vi "Lab Panel V4.87.vi"() -> ()   [LabVIEW 2013] (continued)
              n211 = local read "LAB05 TEMP"() -> (w259:T12)
              n212 = Unbundle By Name(w259) -> ("T1 Live"=w258:dbl, "T1 Neut"=w257:dbl, "T2 Live"=w256:dbl, "T2 Neut"=w255:dbl)  [unwired: 2 out]
              n213 = local read "TEMP LA05"() -> (w260:T9)
              n214 = Bundle By Name(cluster=w260, "TL-1"=w258, "TN-1"=w257, "TL-2"=w256, "TN-2"=w255, "TL -1COUNT"=w253, "TN-1 COUNT"=w253, "TL-2 COUNT"=w253, "TN-2 COUNT"=w253) -> (w254:T9)
              n215 = local write "TEMP LA05"(w254) -> ()
            }
          }
        }
        frame #8 {
          # "enable front panel, all settings done"
          n216 = property on="Tab Control 2" class="TabCtl (strict)"("DisabledEnum"=T16."Enabled" ("Disabled")) -> ()  [unwired: 2 in, 2 out]
          n217 = property on="Tab Control 2" class="TabCtl (strict)"("Value"=0) -> ()  [unwired: 2 in, 2 out]
        }
        frame #9 {
          # "check network directory valid"
          n218 = while {
            stop <- w265 continue-if-true
            w263 = TRUE
            n219 = local read "Network Directory"() -> (w267:path)
            n220 = property on="Tab Control 2" class="TabCtl (strict)"("Value"=5) -> ()  [unwired: 2 in, 2 out]
            n221 = File/Directory Info(path=w267) -> (error out=w268:errorcluster)  [unwired: 1 in, 6 out]
            n222 = Unbundle(w268) -> ("status"=w265:bool)  [unwired: 2 out]
            n223 = case shown="True" w265 {
              frame False {
                n224 = local write "Message"("") -> ()
              }
              frame True {
                "Message" <- "NETWORK DIRECTORY NOT FOUND!!!!"
              }
            }
            n225 = property on="Message" class="Str"("Text.TextColor"=u32 16711680) -> ()  [unwired: 2 in, 2 out]
            n226 = property on="Network Directory" class="Path"("Blinking"=w263) -> ()  [unwired: 2 in, 2 out]
            n227 = property on="Message" class="Str"("Blinking"=w263) -> ()  [unwired: 2 in, 2 out]
          }
        }
        frame #10 {
          w271 = FALSE
          n228 = property on="Message" class="Str"("Blinking"=w271) -> ()  [unwired: 2 in, 2 out]
          n229 = property on="Network Directory" class="Path"("Blinking"=w271) -> ()  [unwired: 2 in, 2 out]
          n230 = property on="Tab Control 2" class="TabCtl (strict)"("Value"=0) -> ()  [unwired: 2 in, 2 out]
        }
      }
    }
    frame #2 {
      n231 = node-c288("loop  delay(mS)") -> (w275:T17)  [unwired: 3 in]
      n232 = timed-loop {
        timing: w275 -> [_]
        timing-out: [_] -> w274
        i -> [w297]
        stop <- "stop" stop-if-true
        n233 = node-c288() -> ()  [unwired: 1 in, 1 out]
        n234 = global write "Global display 1.vi" "stop disp"("stop") -> ()
        n235 = local read "SELECT LAB05-2"() -> (w277:T3)
        n236 = local read "SELECT LAB05-1"() -> (w278:T3)
        n237 = local read "SELECT LAB04-2"() -> (w279:T3)
        n238 = local read "SELECT LAB03-1"() -> (w282:T3)
        n239 = local read "SELECT LAB02-2"() -> (w283:T3)
        n240 = local read "SELECT LAB01-1"() -> (w286:T3)
        n241 = local read "SELECT LAB03-2"() -> (w281:T3)
        n242 = local read "SELECT LAB01-2"() -> (w285:T3)
        n243 = local read "SELECT LAB04-1"() -> (w280:T3)
        n244 = local read "SELECT LAB02-1"() -> (w284:T3)
        n245 = local read "run lab03-2"() -> (w291:bool)
        n246 = local read "run lab04-1"() -> (w290:bool)
        n247 = local read "run lab05-1"() -> (w288:bool)
        n248 = local read "run lab04-2"() -> (w289:bool)
        n249 = local read "run lab05-2"() -> (w287:bool)
        n250 = local read "run lab03-1"() -> (w292:bool)
        n251 = local read "run lab02-2"() -> (w293:bool)
        n252 = local read "run lab02-1"() -> (w294:bool)
        n253 = local read "run lab01-1"() -> (w296:bool)
        n254 = local read "run lab01-2"() -> (w295:bool)
        n255 = stacked-sequence {
          seq-local: [_ w359 _ _ _ _ _ _ _ _ _ _ _ _ _ _ _ _ _ _ _ _ _] -> [_ _ _ _ _ w2438 _ _ _ _ _ _ _ _ _ _ _ _ _ _ _ _ _]
          seq-local: [_ w358 _ _ _ _ _ _ _ _ _ _ _ _ _ _ _ _ _ _ _ _ _] -> [_ _ _ _ _ w2437 _ _ _ _ _ _ _ _ _ _ _ _ _ _ _ _ _]
          seq-local: [_ w345 _ _ _ _ _ _ _ _ _ _ _ _ _ _ _ _ _ _ _ _ _] -> [_ _ _ _ _ w2436 _ _ _ _ _ _ _ _ _ _ _ _ _ _ _ _ _]
          seq-local: [_ w344 _ _ _ _ _ _ _ _ _ _ _ _ _ _ _ _ _ _ _ _ _] -> [_ _ _ _ _ w2435 _ _ _ _ _ _ _ _ _ _ _ _ _ _ _ _ _]
          seq-local: [_ w343 _ _ _ _ _ _ _ _ _ _ _ _ _ _ _ _ _ _ _ _ _] -> [_ _ _ _ _ w2434 _ _ _ _ _ _ _ _ _ _ _ _ _ _ _ _ _]
          seq-local: [_ w342 _ _ _ _ _ _ _ _ _ _ _ _ _ _ _ _ _ _ _ _ _] -> [_ _ _ _ _ w2433 _ _ _ _ _ _ _ _ _ _ _ _ _ _ _ _ _]
          seq-local: [_ w341 _ _ _ _ _ _ _ _ _ _ _ _ _ _ _ _ _ _ _ _ _] -> [_ _ _ _ _ w2432 _ _ _ _ _ _ _ _ _ _ _ _ _ _ _ _ _]
          seq-local: [_ w340 _ _ _ _ _ _ _ _ _ _ _ _ _ _ _ _ _ _ _ _ _] -> [_ _ _ _ _ w2431 _ _ _ _ _ _ _ _ _ _ _ _ _ _ _ _ _]
          seq-local: [_ w339 _ _ _ _ _ _ _ _ _ _ _ _ _ _ _ _ _ _ _ _ _] -> [_ _ _ _ _ w2430 _ _ _ _ _ _ _ _ _ _ _ _ _ _ _ _ _]
          seq-local: [_ w338 _ _ _ _ _ _ _ _ _ _ _ _ _ _ _ _ _ _ _ _ _] -> [_ _ _ _ _ w2429 _ _ _ _ _ _ _ _ _ _ _ _ _ _ _ _ _]
          tunnel: w296 -> [_ _ w375 w621 w2028 w2458 w2773 w3260 _ _ _ _ w3671 _ w4628 _ _ w4913 w5216 w5398 _ _ _]
          tunnel: w295 -> [_ _ w374 w619 w2027 w2457 w2774 w3259 _ _ _ _ w3670 _ w4626 _ _ w4912 w5215 w5396 _ _ _]
          tunnel: w294 -> [_ _ w373 w617 w2026 w2456 w2772 w3258 _ _ _ _ w3669 _ w4624 _ _ w4911 w5214 w5395 _ _ _]
          tunnel: w293 -> [_ _ w372 w615 w2025 w2455 w2771 w3257 _ _ _ _ w3668 _ w4622 _ _ w4910 w5213 w5394 _ _ _]
          tunnel: w292 -> [_ _ w371 w613 w2024 w2454 w2770 w3256 _ _ _ _ w3667 _ w4620 _ _ w4909 w5212 w5393 _ _ _]
          tunnel: w291 -> [_ _ w370 w611 w2023 w2453 w2769 w3255 _ _ _ _ w3666 _ w4618 _ _ w4908 w5211 w5392 _ _ _]
          tunnel: w290 -> [_ _ w369 w609 w2022 w2452 w2768 w3254 _ _ _ _ w3665 _ w4616 _ _ w4907 w5210 w5391 _ _ _]
          tunnel: w289 -> [_ _ w368 w607 w2021 w2451 w2767 w3253 _ _ _ _ w3664 _ w4614 _ _ w4906 w5209 w5390 _ _ _]
          tunnel: w288 -> [_ _ w367 w605 w2020 w2450 w2766 w3252 _ _ _ _ w3663 _ w4612 _ _ w4905 w5208 w5389 _ _ _]
          tunnel: w287 -> [_ _ w366 w603 w2019 w2449 w2765 w3251 _ _ _ _ w3662 _ w4610 _ _ w4904 w5207 w5388 _ _ _]
          tunnel: w286 -> [_ _ _ w620 w2018 w2448 _ _ _ _ _ _ _ _ w4630 _ _ _ _ _ w5736 _ _]
          tunnel: w285 -> [_ _ _ w618 w2017 w2447 _ _ _ _ _ _ _ _ w4625 _ _ _ _ _ w5735 _ _]
          tunnel: w284 -> [_ _ _ w616 w2016 w2446 _ _ _ _ _ _ _ _ w4623 _ _ _ _ _ w5734 _ _]
          tunnel: w283 -> [_ _ _ w614 w2015 w2445 _ _ _ _ _ _ _ _ w4621 _ _ _ _ _ w5733 _ _]
          tunnel: w282 -> [_ _ _ w612 w2014 w2444 _ _ _ _ _ _ _ _ w4619 _ _ _ _ _ w5732 _ _]
          tunnel: w281 -> [_ _ _ w610 w2013 w2443 _ _ _ _ _ _ _ _ w4617 _ _ _ _ _ w5731 _ _]
          tunnel: w280 -> [_ _ _ w608 w2012 w2442 _ _ _ _ _ _ _ _ w4615 _ _ _ _ _ w5730 _ _]
          tunnel: w279 -> [_ _ _ w606 w2011 w2441 _ _ _ _ _ _ _ _ w4613 _ _ _ _ _ w5729 _ _]
          tunnel: w278 -> [_ _ _ w604 w2010 w2440 _ _ _ _ _ _ _ _ w4611 _ _ _ _ _ w5728 _ _]
          tunnel: w277 -> [_ _ _ w602 w2009 w2439 _ _ _ _ _ _ _ _ w4609 _ _ _ _ _ w5727 _ _]
          frame #0 {
            w301 = FALSE
            w306 = 0.5
            # "set up cycle control"
            n256 = local read "jig cycle"() -> (w305:dbl)
            n257 = Divide(x="JIG ON TIME (S)", y=w306) -> (x/y=→"on loops":dbl)
            n258 = Divide(x="JIG OFF TIME (S)", y=w306) -> (x/y=→"off loops":dbl)
            n259 = Increment(x=w305) -> (x+1=w304:dbl)
            n260 = local write "TEMP"(w301) -> ()
            n261 = local write "AI"(w301) -> ()
            n262 = local write "jig cycle"(w304) -> ()
            n263 = event shown="[1] \"ADMIN\": Value Change" {
              selector: _ -> [_ _]
              dyn-events: _ -> [_ _]
              timeout: 10 -> [_ _]
              event Timeout {
                n264 = event-data() -> ()  [unwired: 1 in, 3 out]
              }
              event "ADMIN": Value Change {
                n265 = event-data() -> ()  [unwired: 1 in, 6 out]
                n266 = stacked-sequence {
                  seq-local: [_ w310 _] -> [_ _ w311]
                  frame #0 {
                    n267 = global write "Global 1.vi" "password"("9999") -> ()
                  }
                  frame #1 {
                    n268 = call "sub vi - password 1.vi"() -> ("RESULT"=w310:bool)  [unwired: 11 in]
                  }
                  frame #2 {
                    w313 = FALSE
                    n269 = property on="Tab Control 2" class="TabCtl (strict)"() -> ("Pages"=w317:refnum<vi>[])  [unwired: 2 in, 2 out]
                    n270 = Select(t=TRUE, s=w311, f=w313) -> (s? t:f=w312:bool)
                    n271 = Index Array(array=w317, index=8) -> (element=w315:refnum<vi>)
                    n272 = property class="Page"(reference=w315, "PageVis"=w312) -> ()  [unwired: 1 in, 2 out]
                    n273 = local write "ADMIN"(w313) -> ()
                  }
                }
              }
            }
          }
          frame #1 {
            w355 = 60.0
            # "convert temperature rise minutes to cycles"
            n274 = local read "SET LAB05-2"() -> (w319:T5)
            n275 = local read "SET LAB05-1"() -> (w321:T5)
            n276 = local read "SET LAB04-2"() -> (w323:T5)
            n277 = local read "SET LAB01-1"() -> (w337:T5)
            n278 = local read "SET LAB01-2"() -> (w335:T5)
            n279 = local read "SET LAB02-2"() -> (w331:T5)
            n280 = local read "SET LAB04-1"() -> (w325:T5)
            n281 = local read "SET LAB03-1"() -> (w329:T5)
            n282 = local read "SET LAB03-2"() -> (w327:T5)
            n283 = local read "SET LAB02-1"() -> (w333:T5)
            n284 = local read "JIG OFF TIME (S)"() -> (w360:dbl)
            n285 = local read "JIG ON TIME (S)"() -> (w361:dbl)
            n286 = Unbundle(w319) -> ("T-RISE mins"=w318:dbl)  [unwired: 4 out]
            n287 = Unbundle(w321) -> ("T-RISE mins"=w320:dbl)  [unwired: 4 out]
            n288 = Unbundle(w337) -> ("T-RISE mins"=w336:dbl)  [unwired: 4 out]
            n289 = Unbundle(w323) -> ("T-RISE mins"=w322:dbl)  [unwired: 4 out]
            n290 = Unbundle(w335) -> ("T-RISE mins"=w334:dbl)  [unwired: 4 out]
            n291 = Unbundle(w333) -> ("T-RISE mins"=w332:dbl)  [unwired: 4 out]
            n292 = Unbundle(w325) -> ("T-RISE mins"=w324:dbl)  [unwired: 4 out]
            n293 = Unbundle(w331) -> ("T-RISE mins"=w330:dbl)  [unwired: 4 out]
            n294 = Unbundle(w327) -> ("T-RISE mins"=w326:dbl)  [unwired: 4 out]
            n295 = Unbundle(w329) -> ("T-RISE mins"=w328:dbl)  [unwired: 4 out]
            n296 = Add(x=w361, y=w360) -> (x+y=w354:dbl)
            n297 = Multiply(x=w355, y=w326) -> (x*y=w350:dbl)
            n298 = Multiply(x=w355, y=w324) -> (x*y=w349:dbl)
            n299 = Multiply(x=w355, y=w322) -> (x*y=w348:dbl)
            n300 = Multiply(x=w355, y=w320) -> (x*y=w347:dbl)
            n301 = Multiply(x=w355, y=w318) -> (x*y=w346:dbl)
            n302 = Multiply(x=w355, y=w334) -> (x*y=w356:dbl)
            n303 = Multiply(x=w355, y=w328) -> (x*y=w351:dbl)
            n304 = Multiply(x=w355, y=w336) -> (x*y=w357:dbl)
            n305 = Multiply(x=w355, y=w332) -> (x*y=w353:dbl)
            n306 = Multiply(x=w355, y=w330) -> (x*y=w352:dbl)
            n307 = Divide(x=w347, y=w354) -> (x/y=w339:dbl)
            n308 = Divide(x=w348, y=w354) -> (x/y=w340:dbl)
            n309 = Divide(x=w349, y=w354) -> (x/y=w341:dbl)
            n310 = Divide(x=w346, y=w354) -> (x/y=w338:dbl)
            n311 = Divide(x=w351, y=w354) -> (x/y=w343:dbl)
            n312 = Divide(x=w357, y=w354) -> (x/y=w359:dbl)
            n313 = Divide(x=w356, y=w354) -> (x/y=w358:dbl)
            n314 = Divide(x=w353, y=w354) -> (x/y=w345:dbl)
            n315 = Divide(x=w352, y=w354) -> (x/y=w344:dbl)
            n316 = Divide(x=w350, y=w354) -> (x/y=w342:dbl)
          }
          frame #2 {
            # "control cycle loops"
            n317 = local read "JIG OFF TIME (S)"() -> (w364:dbl)
            n318 = local read "JIG ON TIME (S)"() -> (w363:dbl)
            n319 = local read "jig cycle"() -> (w377:dbl)
            n320 = local read "on loops"() -> (w379:dbl)
            n321 = local read "off loops"() -> (w378:dbl)
            n322 = Add(x=w364, y=w363) -> (x+y=w362:dbl)
            n323 = Add(x=w379, y=w378) -> (x+y=w365:dbl)
            n324 = Greater Or Equal?(x=w377, y=w365) -> (x >= y?=w376:bool)
            n325 = case shown="True" w376 {
              tunnel: w375 -> [_ w412]
              tunnel: w374 -> [_ w411]
              tunnel: w373 -> [_ w410]
              tunnel: w372 -> [_ w409]
              tunnel: w371 -> [_ w408]
              tunnel: w370 -> [_ w407]
              tunnel: w369 -> [_ w406]
              tunnel: w368 -> [_ w405]
              tunnel: w367 -> [_ w404]
              tunnel: w366 -> [_ w403]
              tunnel: w362 -> [_ w402]
              frame False {
              }
              frame True {
                # "increment cycle value and convert cycles to minutes for temp rise"
                n326 = stacked-sequence {
                  frame #0 {
                    n327 = local read "PANEL #"() -> (w415:dbl)
                    n328 = Increment(x=w415) -> (x+1=w414:dbl)
                    n329 = local write "PANEL #"(w414) -> ()
                  }
                  frame #1 {
                    n330 = local read "PANEL #"() -> (w416:dbl)
                    n331 = Greater?(x=w416, y=5) -> (0:w418:bool)
                    n332 = case shown="True" w418 {
                      frame False {
                      }
                      frame True {
                        n333 = local write "PANEL #"(1) -> ()
                      }
                    }
                  }
                }
                n334 = local read "JIG RELAY CYCLES"() -> (w401:T8)
                n335 = Unbundle By Name(w401) -> ("LAB01-1"=w399:dbl, "LAB01-2"=w397:dbl, "LAB02-1"=w395:dbl, "LAB02-2"=w393:dbl, "LAB03-1"=w391:dbl, "LAB03-2"=w389:dbl, "LAB04-1"=w387:dbl, "LAB04-2"=w385:dbl, "LAB05-1"=w383:dbl, "LAB05-2"=w381:dbl)
                n336 = stacked-sequence {
                  tunnel: w412 -> [w430 _ _ _ _ _ _ _ _ _]
                  tunnel: w411 -> [_ w447 _ _ _ _ _ _ _ _]
                  tunnel: w410 -> [_ _ w464 _ _ _ _ _ _ _]
                  tunnel: w409 -> [_ _ _ w481 _ _ _ _ _ _]
                  tunnel: w408 -> [_ _ _ _ w498 _ _ _ _ _]
                  tunnel: w407 -> [_ _ _ _ _ w515 _ _ _ _]
                  tunnel: w406 -> [_ _ _ _ _ _ w532 _ _ _]
                  tunnel: w405 -> [_ _ _ _ _ _ _ w549 _ _]
                  tunnel: w404 -> [_ _ _ _ _ _ _ _ w566 _]
                  tunnel: w403 -> [_ _ _ _ _ _ _ _ _ w583]
                  tunnel: w402 -> [w427 w444 w461 w478 w495 w512 w529 w546 w563 w580]
                  tunnel: w399 -> [w421 _ _ _ _ _ _ _ _ _]
                  tunnel: [w420 _ _ _ _ _ _ _ _ _] -> w398
                  tunnel: w397 -> [_ w438 _ _ _ _ _ _ _ _]
                  tunnel: [_ w437 _ _ _ _ _ _ _ _] -> w396
                  tunnel: w395 -> [_ _ w455 _ _ _ _ _ _ _]
                  tunnel: [_ _ w454 _ _ _ _ _ _ _] -> w394
                  tunnel: w393 -> [_ _ _ w472 _ _ _ _ _ _]
                  tunnel: [_ _ _ w471 _ _ _ _ _ _] -> w392
                  tunnel: w391 -> [_ _ _ _ w489 _ _ _ _ _]
                  tunnel: [_ _ _ _ w488 _ _ _ _ _] -> w390
                  tunnel: w389 -> [_ _ _ _ _ w506 _ _ _ _]
                  tunnel: [_ _ _ _ _ w505 _ _ _ _] -> w388
                  tunnel: w387 -> [_ _ _ _ _ _ w523 _ _ _]
                  tunnel: [_ _ _ _ _ _ w522 _ _ _] -> w386
                  tunnel: w385 -> [_ _ _ _ _ _ _ w540 _ _]
                  tunnel: [_ _ _ _ _ _ _ w539 _ _] -> w384
                  tunnel: w383 -> [_ _ _ _ _ _ _ _ w557 _]
                  tunnel: [_ _ _ _ _ _ _ _ w556 _] -> w382
                  tunnel: w381 -> [_ _ _ _ _ _ _ _ _ w574]
                  tunnel: [_ _ _ _ _ _ _ _ _ w573] -> w380
                  frame #0 {
                    n337 = local read "DISP LAB01-1"() -> (w425:T4)
                    n338 = Unbundle(w425) -> ("CYCLE"=w426:dbl)  [unwired: 2 out]
                    n339 = case shown="True" w430 {
                      tunnel: w426 -> [w432 w436]
                      tunnel: [w432 w435] -> w424
                      tunnel: w421 -> [w431 w434]
                      tunnel: [w431 w433] -> w420
                      frame False {
                      }
                      frame True {
                        n340 = Increment(x=w434) -> (x+1=w433:dbl)
                        n341 = Increment(x=w436) -> (x+1=w435:dbl)
                      }
                    }
                    n342 = Multiply(x=w424, y=w427) -> (x*y=w428:dbl)
                    n343 = Divide(x=w428, y=60.0) -> (x/y=w423:dbl)
                    n344 = Bundle(cluster=w425, "CYCLE"=w424, "MINS"=w423) -> (w422:T4)  [unwired: 1 in]
                    n345 = local write "DISP LAB01-1"(w422) -> ()
                  }
                  frame #1 {
                    n346 = local read "DISP LAB01-2"() -> (w442:T4)
                    n347 = Unbundle(w442) -> ("CYCLE"=w443:dbl)  [unwired: 2 out]
                    n348 = case shown="True" w447 {
                      tunnel: w443 -> [w449 w453]
                      tunnel: [w449 w452] -> w440
                      tunnel: w438 -> [w448 w451]
                      tunnel: [w448 w450] -> w437
                      frame False {
                      }
                      frame True {
                        n349 = Increment(x=w451) -> (x+1=w450:dbl)
                        n350 = Increment(x=w453) -> (x+1=w452:dbl)
                      }
                    }
                    n351 = Multiply(x=w440, y=w444) -> (x*y=w445:dbl)
                    n352 = Divide(x=w445, y=60.0) -> (x/y=w439:dbl)
                    n353 = Bundle(cluster=w442, "CYCLE"=w440, "MINS"=w439) -> (w441:T4)  [unwired: 1 in]
                    n354 = local write "DISP LAB01-2"(w441) -> ()
                  }
                  frame #2 {
                    n355 = local read "DISP LAB02-1"() -> (w459:T4)
                    n356 = Unbundle(w459) -> ("CYCLE"=w460:dbl)  [unwired: 2 out]
                    n357 = case shown="True" w464 {
                      tunnel: [w466 w470] -> w457
                      tunnel: w460 -> [w466 w469]
                      tunnel: w455 -> [w465 w468]
                      tunnel: [w465 w467] -> w454
                      frame False {
                      }
                      frame True {
                        n358 = Increment(x=w468) -> (x+1=w467:dbl)
                        n359 = Increment(x=w469) -> (x+1=w470:dbl)
                      }
                    }
                    n360 = Multiply(x=w457, y=w461) -> (x*y=w462:dbl)
                    n361 = Divide(x=w462, y=60.0) -> (x/y=w456:dbl)
                    n362 = Bundle(cluster=w459, "CYCLE"=w457, "MINS"=w456) -> (w458:T4)  [unwired: 1 in]
                    n363 = local write "DISP LAB02-1"(w458) -> ()
                  }
                  frame #3 {
                    n364 = local read "DISP LAB02-2"() -> (w476:T4)
                    n365 = Unbundle(w476) -> ("CYCLE"=w477:dbl)  [unwired: 2 out]
                    n366 = case shown="True" w481 {
                      tunnel: [w483 w487] -> w475
                      tunnel: w477 -> [w483 w486]
                      tunnel: w472 -> [w482 w485]
                      tunnel: [w482 w484] -> w471
                      frame False {
                      }
                      frame True {
                        n367 = Increment(x=w485) -> (x+1=w484:dbl)
                        n368 = Increment(x=w486) -> (x+1=w487:dbl)
                      }
                    }
                    n369 = Multiply(x=w475, y=w478) -> (x*y=w479:dbl)
                    n370 = Divide(x=w479, y=60.0) -> (x/y=w474:dbl)
                    n371 = Bundle(cluster=w476, "CYCLE"=w475, "MINS"=w474) -> (w473:T4)  [unwired: 1 in]
                    n372 = local write "DISP LAB02-2"(w473) -> ()
                  }
                  frame #4 {
                    n373 = local read "DISP LAB03-1"() -> (w493:T4)
                    n374 = Unbundle(w493) -> ("CYCLE"=w494:dbl)  [unwired: 2 out]
                    n375 = case shown="True" w498 {
                      tunnel: [w500 w504] -> w490
                      tunnel: w494 -> [w500 w503]
                      tunnel: w489 -> [w499 w502]
                      tunnel: [w499 w501] -> w488
                      frame False {
                      }
                      frame True {
                        n376 = Increment(x=w502) -> (x+1=w501:dbl)
                        n377 = Increment(x=w503) -> (x+1=w504:dbl)
                      }
                    }
                    n378 = Multiply(x=w490, y=w495) -> (x*y=w496:dbl)
                    n379 = Divide(x=w496, y=60.0) -> (x/y=w491:dbl)
                    n380 = Bundle(cluster=w493, "CYCLE"=w490, "MINS"=w491) -> (w492:T4)  [unwired: 1 in]
                    n381 = local write "DISP LAB03-1"(w492) -> ()
                  }
                  frame #5 {
                    n382 = local read "DISP LAB03-2"() -> (w510:T4)
                    n383 = Unbundle(w510) -> ("CYCLE"=w511:dbl)  [unwired: 2 out]
                    n384 = case shown="True" w515 {
                      tunnel: [w517 w521] -> w509
                      tunnel: w511 -> [w517 w520]
                      tunnel: w506 -> [w516 w519]
                      tunnel: [w516 w518] -> w505
                      frame False {
                      }
                      frame True {
                        n385 = Increment(x=w519) -> (x+1=w518:dbl)
                        n386 = Increment(x=w520) -> (x+1=w521:dbl)
                      }
                    }
                    n387 = Multiply(x=w509, y=w512) -> (x*y=w513:dbl)
                    n388 = Divide(x=w513, y=60.0) -> (x/y=w508:dbl)
                    n389 = Bundle(cluster=w510, "CYCLE"=w509, "MINS"=w508) -> (w507:T4)  [unwired: 1 in]
                    n390 = local write "DISP LAB03-2"(w507) -> ()
                  }
                  frame #6 {
                    n391 = local read "DISP LAB04-1"() -> (w527:T4)
                    n392 = Unbundle(w527) -> ("CYCLE"=w528:dbl)  [unwired: 2 out]
                    n393 = case shown="True" w532 {
                      tunnel: [w534 w538] -> w525
                      tunnel: w528 -> [w534 w537]
                      tunnel: w523 -> [w533 w536]
                      tunnel: [w533 w535] -> w522
                      frame False {
                      }
                      frame True {
                        n394 = Increment(x=w536) -> (x+1=w535:dbl)
                        n395 = Increment(x=w537) -> (x+1=w538:dbl)
                      }
                    }
                    n396 = Multiply(x=w525, y=w529) -> (x*y=w530:dbl)
                    n397 = Divide(x=w530, y=60.0) -> (x/y=w524:dbl)
                    n398 = Bundle(cluster=w527, "CYCLE"=w525, "MINS"=w524) -> (w526:T4)  [unwired: 1 in]
                    n399 = local write "DISP LAB04-1"(w526) -> ()
                  }
                  frame #7 {
                    n400 = local read "DISP LAB04-2"() -> (w544:T4)
                    n401 = Unbundle(w544) -> ("CYCLE"=w545:dbl)  [unwired: 2 out]
                    n402 = case shown="True" w549 {
                      tunnel: [w551 w555] -> w542
                      tunnel: w545 -> [w551 w554]
                      tunnel: w540 -> [w550 w553]
                      tunnel: [w550 w552] -> w539
                      frame False {
                      }
                      frame True {
                        n403 = Increment(x=w553) -> (x+1=w552:dbl)
                        n404 = Increment(x=w554) -> (x+1=w555:dbl)
                      }
                    }
                    n405 = Multiply(x=w542, y=w546) -> (x*y=w548:dbl)
                    n406 = Divide(x=w548, y=60.0) -> (x/y=w541:dbl)
                    n407 = Bundle(cluster=w544, "CYCLE"=w542, "MINS"=w541) -> (w543:T4)  [unwired: 1 in]
                    n408 = local write "DISP LAB04-2"(w543) -> ()
                  }
                  frame #8 {
                    n409 = local read "DISP LAB05-1"() -> (w561:T4)
                    n410 = Unbundle(w561) -> ("CYCLE"=w562:dbl)  [unwired: 2 out]
                    n411 = case shown="True" w566 {
                      tunnel: [w568 w572] -> w559
                      tunnel: w562 -> [w568 w571]
                      tunnel: w557 -> [w567 w570]
                      tunnel: [w567 w569] -> w556
                      frame False {
                      }
                      frame True {
                        n412 = Increment(x=w570) -> (x+1=w569:dbl)
                        n413 = Increment(x=w571) -> (x+1=w572:dbl)
                      }
                    }
                    n414 = Multiply(x=w559, y=w563) -> (x*y=w564:dbl)
                    n415 = Divide(x=w564, y=60.0) -> (x/y=w558:dbl)
                    n416 = Bundle(cluster=w561, "CYCLE"=w559, "MINS"=w558) -> (w560:T4)  [unwired: 1 in]
                    n417 = local write "DISP LAB05-1"(w560) -> ()
                  }
                  frame #9 {
                    n418 = local read "DISP LAB05-2"() -> (w579:T4)
                    n419 = Unbundle(w579) -> ("CYCLE"=w578:dbl)  [unwired: 2 out]
                    n420 = case shown="True" w583 {
                      tunnel: [w585 w589] -> w577
                      tunnel: w578 -> [w585 w588]
                      tunnel: w574 -> [w584 w587]
                      tunnel: [w584 w586] -> w573
                      frame False {
                      }
                      frame True {
                        n421 = Increment(x=w587) -> (x+1=w586:dbl)
                        n422 = Increment(x=w588) -> (x+1=w589:dbl)
                      }
                    }
                    n423 = Multiply(x=w577, y=w580) -> (x*y=w581:dbl)
                    n424 = Divide(x=w581, y=60.0) -> (x/y=w576:dbl)
                    n425 = Bundle(cluster=w579, "CYCLE"=w577, "MINS"=w576) -> (w575:T4)  [unwired: 1 in]
                    n426 = local write "DISP LAB05-2"(w575) -> ()
                  }
                }
                n427 = local write "jig cycle"(0) -> ()
                n428 = Bundle By Name(cluster=w401, "LAB01-1"=w398, "LAB01-2"=w396, "LAB02-1"=w394, "LAB02-2"=w392, "LAB03-1"=w390, "LAB03-2"=w388, "LAB04-1"=w386, "LAB04-2"=w384, "LAB05-1"=w382, "LAB05-2"=w380) -> (w400:T8)
                n429 = local write "JIG RELAY CYCLES"(w400) -> ()
              }
            }
          }
          frame #3 {
            # "START & STOP test RUN switch change, start test if true and stop test if false"
            n430 = Get Date/Time In Seconds() -> (seconds since 1Jan1904=w600:timestamp)
            n431 = local read "C drive data root dir"() -> (w593:path)
            n432 = Format Date/Time String(time format string (%c)="%b\\%a%d", seconds (now)=w600) -> (date/time string=w624:string)  [unwired: 1 in]
            n433 = Format Date/Time String(time format string (%c)="%H%M", seconds (now)=w600) -> (date/time string=w622:string)  [unwired: 1 in]
            n434 = Format Date/Time String(time format string (%c)="LabPanel%Y", seconds (now)=w600) -> (date/time string=w599:string)  [unwired: 1 in]
            n435 = Path To String(path=w593) -> (string=w596:string)
            n436 = global write "Global 1.vi" "C drive root path"(w593) -> ()
            n437 = Concatenate Strings(w596, "\\") -> (w594:string)
            n438 = event shown="[10] \"RUN LAB05-2\": Value Change" {
              selector: _ -> [_ _ _ _ _ _ _ _ _ _ _]
              dyn-events: _ -> [_ _ _ _ _ _ _ _ _ _ _]
              timeout: 10 -> [_ _ _ _ _ _ _ _ _ _ _]
              tunnel: w594 -> [_ w636 w774 w913 w1051 w1189 w1327 w1465 w1603 w1741 w1880]
              tunnel: w624 -> [_ w635 w773 w912 w1050 w1188 w1326 w1464 w1602 w1740 w1879]
              tunnel: w622 -> [_ w633 w772 w911 w1049 w1187 w1325 w1463 w1601 w1739 w1878]
              tunnel: w620 -> [_ w634 _ _ _ _ _ _ _ _ _]
              tunnel: w621 -> [_ _ _ _ _ _ _ _ _ _ _]
              tunnel: w619 -> [_ _ _ _ _ _ _ _ _ _ _]
              tunnel: w618 -> [_ _ w771 _ _ _ _ _ _ _ _]
              tunnel: w617 -> [_ _ _ _ _ _ _ _ _ _ _]
              tunnel: w616 -> [_ _ _ w910 _ _ _ _ _ _ _]
              tunnel: w615 -> [_ _ _ _ _ _ _ _ _ _ _]
              tunnel: w614 -> [_ _ _ _ w1048 _ _ _ _ _ _]
              tunnel: w613 -> [_ _ _ _ _ _ _ _ _ _ _]
              tunnel: w612 -> [_ _ _ _ _ w1186 _ _ _ _ _]
              tunnel: w611 -> [_ _ _ _ _ _ _ _ _ _ _]
              tunnel: w610 -> [_ _ _ _ _ _ w1324 _ _ _ _]
              tunnel: w609 -> [_ _ _ _ _ _ _ _ _ _ _]
              tunnel: w608 -> [_ _ _ _ _ _ _ w1462 _ _ _]
              tunnel: w607 -> [_ _ _ _ _ _ _ _ _ _ _]
              tunnel: w606 -> [_ _ _ _ _ _ _ _ w1600 _ _]
              tunnel: w605 -> [_ _ _ _ _ _ _ _ _ _ _]
              tunnel: w604 -> [_ _ _ _ _ _ _ _ _ w1738 _]
              tunnel: w603 -> [_ _ _ _ _ _ _ _ _ _ _]
              tunnel: w602 -> [_ _ _ _ _ _ _ _ _ _ w1877]
              tunnel: w599 -> [_ w632 w770 w909 w1047 w1185 w1323 w1461 w1599 w1737 w1876]
              tunnel: [_ w631 w769 w908 w1046 w1184 w1322 w1460 w1598 w1736 w1875] -> w597
              tunnel: "RESET CYCLES TO ZERO?" -> [_ w630 w767 w906 w1044 w1182 w1320 w1458 w1596 w1734 w1873]
              tunnel: "YES" -> [_ w629 w766 w905 w1043 w1181 w1319 w1457 w1595 w1733 w1872]
              tunnel: "NO" -> [_ w628 w765 w904 w1042 w1180 w1318 w1456 w1594 w1732 w1871]
              event Timeout {
                n439 = event-data() -> ()  [unwired: 1 in, 3 out]
              }
              event "RUN LAB01-1": Value Change {
                n440 = event-data() -> ("NewVal"=w626:bool)  [unwired: 1 in, 5 out]
                n441 = local read "SIG LAB01-1"() -> (w627:T2)
                n442 = local write "run lab01-1"(w626) -> ()
                n443 = case shown="True" w626 {
                  tunnel: w636 -> [_ w673]
                  tunnel: w635 -> [_ w672]
                  tunnel: w634 -> [w638 w671]
                  tunnel: w633 -> [_ w670]
                  tunnel: w632 -> [_ w669]
                  tunnel: [w637 w668] -> w631
                  tunnel: w630 -> [_ w667]
                  tunnel: w629 -> [_ w666]
                  tunnel: w628 -> [_ w665]
                  tunnel: w627 -> [_ w664]
                  frame False {
                    # "stop test"
                    n444 = stacked-sequence {
                      tunnel: w638 -> [_ w650 _]
                      tunnel: [_ w642 _] -> w637
                      frame #0 {
                        n445 = local read "DISP LAB01-1"() -> (w641:T4)
                        n446 = Bundle(cluster=w641, "STATUS"="STOP") -> (w639:T4)  [unwired: 2 in]
                        n447 = local write "DISP LAB01-1"(w639) -> ()
                      }
                      frame #1 {
                        n448 = local read "DISP LAB01-1"() -> (w649:T4)
                        n449 = Unbundle(w649) -> ("CYCLE"=w647:dbl, "MINS"=w648:dbl)  [unwired: 1 out]
                        n450 = case shown="\"CYCLE TEST\"" w650 {
                          tunnel: w648 -> [_ _ w657]
                          tunnel: w647 -> [w655 w656 _]
                          tunnel: [w655 w656 w657] -> w646
                          frame "CHART TEST", Default {
                          }
                          frame "CYCLE TEST" {
                          }
                          frame "T-RISE TEST" {
                          }
                        }
                        n451 = local read "TDMS LAB01-1"() -> (w654:refnum<k34>)
                        n452 = Build Array("STOPPED") -> (w651:string[])
                        n453 = Build Array(w646) -> (w645:dbl[])
                        n454 = TDMS Write(0:w654, 5:"TEST RESULT", 7:w651, 9:w645) -> (4:w643:refnum<k34>, 15:w644:errorcluster)  [unwired: 2 in, 2 out]
                        n455 = TDMS Close(8:w644, 11:w643) -> (0:w642:errorcluster)  [unwired: 1 out]
                      }
                      frame #2 {
                        n456 = stacked-sequence {
                          tunnel: "LAB01-1" -> [w660 w662]
                          frame #0 {
                            n457 = call "sub vi - defrag tdms v1.vi"("panel id"=w660) -> ("error out"=w659:errorcluster)  [unwired: 10 in]
                            n458 = local write "data file error"(w659) -> ()
                          }
                          frame #1 {
                            n459 = call "Save data file to network drive v2.vi"("panel id"=w662) -> ("network file save error"=w661:errorcluster)  [unwired: 9 in, 1 out]
                            n460 = local write "RESULT LAB01-1"(FALSE) -> ()
                            n461 = local write "data file error"(w661) -> ()
                          }
                        }
                      }
                    }
                  }
                  frame True {
                    n462 = stacked-sequence {
                      seq-local: [w675 _] -> [_ w678]
                      tunnel: w673 -> [_ w688]
                      tunnel: w672 -> [_ w687]
                      tunnel: w671 -> [_ w686]
                      tunnel: w670 -> [_ w685]
                      tunnel: w669 -> [_ w684]
                      tunnel: [_ w683] -> w668
                      tunnel: w667 -> [_ w682]
                      tunnel: w666 -> [_ w681]
                      tunnel: w665 -> [_ w680]
                      tunnel: w664 -> [w677 w679]
                      frame #0 {
                        n463 = Unbundle(w677) -> ("AMPS"=w676:dbl)  [unwired: 4 out]
                        n464 = call "Check For Amps on v1.vi"("ID"="LAB01-1", "amps"=w676) -> ("amps"=w675:bool)  [unwired: 9 in]
                      }
                      frame #1 {
                        n465 = case shown="True" w678 {
                          tunnel: w688 -> [_ w700]
                          tunnel: w687 -> [_ w699]
                          tunnel: w686 -> [_ w698]
                          tunnel: w685 -> [_ w697]
                          tunnel: w684 -> [_ w696]
                          tunnel: [errorcluster {"status"=FALSE, "code"=0, "source"=""} ("error out") w695] -> w683
                          tunnel: w682 -> [_ w694]
                          tunnel: w681 -> [_ w693]
                          tunnel: w680 -> [_ w692]
                          tunnel: w679 -> [_ w691]
                          frame False {
                            w689 = FALSE
                            n466 = local write "RUN LAB01-1"(w689) -> ()
                            n467 = local write "run lab01-1"(w689) -> ()
                          }
                          frame True {
                            n468 = stacked-sequence {
                              seq-local: [w701 _ _ _ _] -> [_ w722 _ _ _]
                              tunnel: w700 -> [w706 _ _ _ _]
                              tunnel: w699 -> [w702 _ _ _ _]
                              tunnel: w698 -> [w716 _ _ _ _]
                              tunnel: w697 -> [w709 _ _ _ _]
                              tunnel: w696 -> [w704 _ _ _ _]
                              tunnel: [_ w723 _ _ _] -> w695
                              tunnel: w694 -> [_ _ _ w744 _]
                              tunnel: w693 -> [_ _ _ w754 _]
                              tunnel: w692 -> [_ _ _ w753 _]
                              tunnel: w691 -> [_ _ _ _ w760]
                              frame #0 {
                                w703 = "\\"
                                n469 = case shown="\"CHART TEST\", Default" w716 {
                                tunnel: ["L01-1-CHART TEST-" "L01-1-CYCLE TEST-" "L01-1-T-RISE TEST-"] -> w712
                                frame "CHART TEST", Default {
                                }
                                frame "CYCLE TEST" {
                                }
                                frame "T-RISE TEST" {
                                }
                                }
                                n470 = local read "SET LAB01-1"() -> (w711:T5)
                                n471 = Unbundle(w711) -> ("DESCRIPTION"=w710:string)  [unwired: 4 out]
                                n472 = Concatenate Strings(w706, "\\", w704, w703, w702, w703) -> (w713:string)
                                n473 = String To Path(string=w713) -> (path=w715:path)
                                n474 = Concatenate Strings(w713, w712, w710, "-", w709, ".tdms") -> (w701:string)
                                n475 = Create Folder(path (use dialog)=w715) -> (error out=w714:errorcluster)  [unwired: 2 in, 2 out]
                                n476 = call <vilib>:"Clear Errors.vi"("error in (no error)"=w714) -> ()  [unwired: 6 in, 1 out]
                                n477 = global write "Global 1.vi" "LAB01-1 FILE"(w701) -> ()
                              }
                              frame #1 {
                                (unwired) FALSE
                                n478 = String To Path(string=w722) -> (path=w720:path)
                                n479 = TDMS Open(6:FALSE, 10:T20."create or replace" ("operation (0:open)"), 11:w720) -> (0:w723:errorcluster, 3:→"TDMS LAB01-1":refnum<k34>)  [unwired: 4 in]
                              }
                              frame #2 {
                                n480 = local read "TDMS LAB01-1"() -> (w742:refnum<k34>)
                                n481 = local read "SET LAB01-1"() -> (w731:T5)
                                n482 = Build Array("Testers Name", "Description", "Set Test Cycles", "T-Rise minutes", "T-Rise Deg C") -> (w732:string[])
                                n483 = Unbundle(w731) -> ("NAME"=w730:string, "DESCRIPTION"=w729:string, "CYCLES"=w728:dbl, "T-RISE mins"=w727:dbl, "T-RISE deg C"=w726:dbl)
                                n484 = Number To Decimal String(number=w728) -> (decimal integer string=w741:string)  [unwired: 1 in]
                                n485 = Number To Decimal String(number=w727) -> (decimal integer string=w740:string)  [unwired: 1 in]
                                n486 = Number To Decimal String(number=w726) -> (decimal integer string=w739:string)  [unwired: 1 in]
                                n487 = Build Array(w730, w729, w741, w740, w739) -> (w738:string[])
                                n488 = TDMS Set Properties(5:w738, 7:w732, 11:w742) -> ()  [unwired: 3 in, 4 out]
                              }
                              frame #3 {
                                n489 = local read "DISP LAB01-1"() -> (w752:T4)
                                n490 = Concatenate Strings("LAB01-1  ", w744) -> (w743:string)
                                n491 = Two Button Dialog(message=w743, 1:w753, 2:w754) -> (T button?=w746:bool)
                                n492 = case shown="True" w746 {
                                tunnel: w752 -> [w757 w758]
                                tunnel: [w757 w758] -> w751
                                tunnel: [w756 w759] -> w750
                                tunnel: [w755 w759] -> w749
                                frame False {
                                n493 = Unbundle(w757) -> ("CYCLE"=w756:dbl, "MINS"=w755:dbl)  [unwired: 1 out]
                                }
                                frame True {
                                w759 = 0.0
                                }
                                }
                                n494 = Bundle(cluster=w751, "CYCLE"=w750, "MINS"=w749, "STATUS"="RUN") -> (w748:T4)
                                n495 = local write "DISP LAB01-1"(w748) -> ()
                              }
                              frame #4 {
                                n496 = local read "TEMP START LAB01-1"() -> (w764:cluster{"TL":dbl, "TN":dbl})
                                n497 = Unbundle(w760) -> ("Tmp Live"=w762:dbl, "Tmp Neut"=w761:dbl)  [unwired: 3 out]
                                n498 = Bundle(cluster=w764, "TL"=w762, "TN"=w761) -> (w763:cluster{"TL":dbl, "TN":dbl})
                                n499 = local write "TEMP START LAB01-1"(w763) -> ()
                              }
                            }
                          }
                        }
                      }
                    }
                  }
                }
              }
              event "RUN LAB01-2": Value Change {
                n500 = event-data() -> ("NewVal"=w768:bool)  [unwired: 1 in, 5 out]
                n501 = local write "run lab01-2"(w768) -> ()
                n502 = case shown="True" w768 {
                  tunnel: w774 -> [_ w811]
                  tunnel: w773 -> [_ w810]
                  tunnel: w771 -> [w776 w809]
                  tunnel: w772 -> [_ w808]
                  tunnel: w770 -> [_ w807]
                  tunnel: [w775 w806] -> w769
                  tunnel: w767 -> [_ w805]
                  tunnel: w766 -> [_ w804]
                  tunnel: w765 -> [_ w803]
                  frame False {
                    # "stop test"
                    n503 = stacked-sequence {
                      tunnel: w776 -> [w785 _]
                      tunnel: [w777 _] -> w775
                      frame #0 {
                        n504 = local read "DISP LAB01-2"() -> (w784:T4)
                        n505 = Unbundle(w784) -> ("CYCLE"=w782:dbl, "MINS"=w783:dbl)  [unwired: 1 out]
                        n506 = case shown="\"CHART TEST\", Default" w785 {
                          tunnel: w783 -> [_ _ w792]
                          tunnel: w782 -> [w790 w791 _]
                          tunnel: [w790 w791 w792] -> w781
                          frame "CHART TEST", Default {
                          }
                          frame "CYCLE TEST" {
                          }
                          frame "T-RISE TEST" {
                          }
                        }
                        n507 = local read "TDMS LAB01-2"() -> (w789:refnum<k34>)
                        n508 = Build Array("STOPPED") -> (w786:string[])
                        n509 = Build Array(w781) -> (w780:dbl[])
                        n510 = TDMS Write(0:w789, 5:"TEST RESULT", 7:w786, 9:w780) -> (4:w778:refnum<k34>, 15:w779:errorcluster)  [unwired: 2 in, 2 out]
                        n511 = TDMS Close(8:w779, 11:w778) -> (0:w777:errorcluster)  [unwired: 1 out]
                      }
                      frame #1 {
                        n512 = local read "DISP LAB01-2"() -> (w796:T4)
                        n513 = stacked-sequence {
                          tunnel: "LAB01-2" -> [w798 w800]
                          frame #0 {
                            n514 = call "sub vi - defrag tdms v1.vi"("panel id"=w798) -> ("error out"=w797:errorcluster)  [unwired: 10 in]
                            n515 = local write "data file error"(w797) -> ()
                          }
                          frame #1 {
                            n516 = call "Save data file to network drive v2.vi"("panel id"=w800) -> ("network file save error"=w799:errorcluster)  [unwired: 9 in, 1 out]
                            n517 = local write "RESULT LAB01-2"(FALSE) -> ()
                            n518 = local write "data file error"(w799) -> ()
                          }
                        }
                        n519 = Bundle(cluster=w796, "STATUS"="STOP") -> (w794:T4)  [unwired: 2 in]
                        n520 = local write "DISP LAB01-2"(w794) -> ()
                      }
                    }
                  }
                  frame True {
                    n521 = local read "SIG LAB01-2"() -> (w802:T2)
                    n522 = stacked-sequence {
                      seq-local: [w813 _] -> [_ w816]
                      tunnel: w811 -> [_ w826]
                      tunnel: w810 -> [_ w825]
                      tunnel: w809 -> [_ w824]
                      tunnel: w808 -> [_ w823]
                      tunnel: w807 -> [_ w822]
                      tunnel: [_ w821] -> w806
                      tunnel: w805 -> [_ w820]
                      tunnel: w804 -> [_ w819]
                      tunnel: w803 -> [_ w818]
                      tunnel: w802 -> [w812 w817]
                      frame #0 {
                        n523 = Unbundle(w812) -> ("AMPS"=w815:dbl)  [unwired: 4 out]
                        n524 = call "Check For Amps on v1.vi"("ID"="LAB01-2", "amps"=w815) -> ("amps"=w813:bool)  [unwired: 9 in]
                      }
                      frame #1 {
                        n525 = case shown="True" w816 {
                          tunnel: w826 -> [_ w838]
                          tunnel: w825 -> [_ w837]
                          tunnel: w824 -> [_ w836]
                          tunnel: w823 -> [_ w835]
                          tunnel: w822 -> [_ w834]
                          tunnel: [errorcluster {"status"=FALSE, "code"=0, "source"=""} ("error out") w833] -> w821
                          tunnel: w820 -> [_ w832]
                          tunnel: w819 -> [_ w831]
                          tunnel: w818 -> [_ w830]
                          tunnel: w817 -> [_ w829]
                          frame False {
                            w827 = FALSE
                            n526 = local write "RUN LAB01-2"(w827) -> ()
                            n527 = local write "run lab01-2"(w827) -> ()
                          }
                          frame True {
                            n528 = stacked-sequence {
                              seq-local: [w839 _ _ _ _] -> [_ w863 _ _ _]
                              tunnel: w838 -> [w844 _ _ _ _]
                              tunnel: w837 -> [w841 _ _ _ _]
                              tunnel: w836 -> [w854 _ _ _ _]
                              tunnel: w835 -> [w847 _ _ _ _]
                              tunnel: w834 -> [w842 _ _ _ _]
                              tunnel: [_ w858 _ _ _] -> w833
                              tunnel: w832 -> [_ _ _ w885 _]
                              tunnel: w831 -> [_ _ _ w884 _]
                              tunnel: w830 -> [_ _ _ w883 _]
                              tunnel: w829 -> [_ _ _ _ w898]
                              frame #0 {
                                w840 = "\\"
                                n529 = local read "SET LAB01-2"() -> (w849:T5)
                                n530 = case shown="\"CYCLE TEST\"" w854 {
                                tunnel: ["L01-2-CHART TEST-" "L01-2-CYCLE TEST-" "L01-2-T-RISE TEST-"] -> w850
                                frame "CHART TEST", Default {
                                }
                                frame "CYCLE TEST" {
                                }
                                frame "T-RISE TEST" {
                                }
                                }
                                n531 = Unbundle(w849) -> ("DESCRIPTION"=w848:string)  [unwired: 4 out]
                                n532 = Concatenate Strings(w844, "\\", w842, w840, w841, w840) -> (w851:string)
                                n533 = String To Path(string=w851) -> (path=w853:path)
                                n534 = Concatenate Strings(w851, w850, w848, "-", w847, ".tdms") -> (w839:string)
                                n535 = Create Folder(path (use dialog)=w853) -> (error out=w852:errorcluster)  [unwired: 2 in, 2 out]
                                n536 = call <vilib>:"Clear Errors.vi"("error in (no error)"=w852) -> ()  [unwired: 6 in, 1 out]
                                n537 = global write "Global 1.vi" "LAB01-2 FILE"(w839) -> ()
                              }
                              frame #1 {
                                (unwired) FALSE
                                n538 = String To Path(string=w863) -> (path=w859:path)
                                n539 = TDMS Open(6:FALSE, 10:T20."create or replace" ("operation (0:open)"), 11:w859) -> (0:w858:errorcluster, 3:→"TDMS LAB01-2":refnum<k34>)  [unwired: 4 in]
                              }
                              frame #2 {
                                n540 = local read "SET LAB01-2"() -> (w869:T5)
                                n541 = local read "TDMS LAB01-2"() -> (w880:refnum<k34>)
                                n542 = Build Array("Testers Name", "Description", "Set Test Cycles", "T-Rise minutes", "T-Rise Deg C") -> (w870:string[])
                                n543 = Unbundle(w869) -> ("NAME"=w868:string, "DESCRIPTION"=w867:string, "CYCLES"=w866:dbl, "T-RISE mins"=w865:dbl, "T-RISE deg C"=w864:dbl)
                                n544 = Number To Decimal String(number=w866) -> (decimal integer string=w879:string)  [unwired: 1 in]
                                n545 = Number To Decimal String(number=w865) -> (decimal integer string=w878:string)  [unwired: 1 in]
                                n546 = Number To Decimal String(number=w864) -> (decimal integer string=w877:string)  [unwired: 1 in]
                                n547 = Build Array(w868, w867, w879, w878, w877) -> (w876:string[])
                                n548 = TDMS Set Properties(5:w876, 7:w870, 11:w880) -> ()  [unwired: 3 in, 4 out]
                              }
                              frame #3 {
                                n549 = local read "DISP LAB01-2"() -> (w882:T4)
                                n550 = Concatenate Strings("LAB01-2  ", w885) -> (w886:string)
                                n551 = Two Button Dialog(message=w886, 1:w883, 2:w884) -> (T button?=w888:bool)
                                n552 = case shown="True" w888 {
                                tunnel: w882 -> [w895 w896]
                                tunnel: [w895 w896] -> w892
                                tunnel: [w894 w897] -> w891
                                tunnel: [w893 w897] -> w890
                                frame False {
                                n553 = Unbundle(w895) -> ("CYCLE"=w894:dbl, "MINS"=w893:dbl)  [unwired: 1 out]
                                }
                                frame True {
                                w897 = 0.0
                                }
                                }
                                n554 = Bundle(cluster=w892, "CYCLE"=w891, "MINS"=w890, "STATUS"="RUN") -> (w881:T4)
                                n555 = local write "DISP LAB01-2"(w881) -> ()
                              }
                              frame #4 {
                                n556 = local read "TEMP START LAB01-2"() -> (w902:cluster{"TL":dbl, "TN":dbl})
